vi "ChipKit Stepper Motor.vi"() -> ()   [LabVIEW 2011, in "LabVIEW Interface for ChipKit.lvlib"]
doc: "This example shows how to use the ChipKit's Stepper Motor API. The fritzing diagram shows use with the EasyStepper 4.3 or 4.4 motor controller."
uses:
  vi.lib/LabVIEW Interface for ChipKit/LabVIEW Interface for ChipKit.lvlib
panel:
  in  "VISA resource name":refnum<visa-resource-name>
  in  "Stop":bool
  in  "Stepper #":u8=1
  in  "OK Button":bool
  in  "Set Acceleration (0 to disable)":i16
  in  "# of Steps to Move":i16
  in  "Set Speed (Steps per Second)":i16=100
  out "Steps Remaining?":bool
  in  "Dial":i16(knob) scale=0.0..200.0
  in  "error in":errorcluster
  # "Preset Movement"
  # "Interactive Movement"
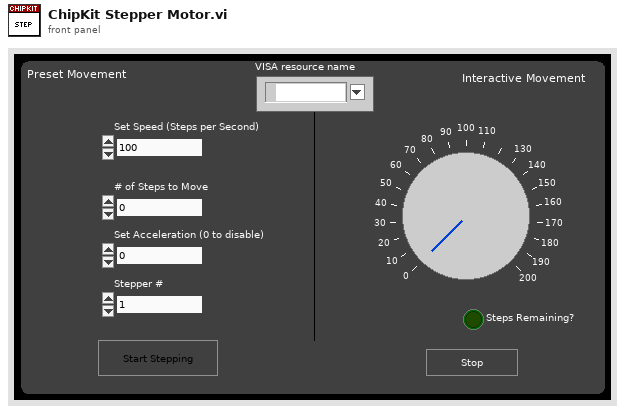
[diagram p1: front panel]
types:
  T1 = typedef "LabVIEW Interface for ChipKit.lvlib/Chipkit Resource.ctl" = cluster{"VISA resource":refnum<visa-resource-name>, "Board Type":T2, "Connection Type":enum8{"USB / Serial"}, "Bytes Per Packet (15)":u8}
  T2 = typedef "LabVIEW Interface for ChipKit.lvlib/Board Type.ctl" = enum16{"Arduino Uno", "Dimuelanove w/Atmega 328", "Mega 2560", "Chipkit Uno32", "Chipkit Max32"}
  T3 = typedef "LabVIEW Interface for ChipKit.lvlib/Chipkit Resource.ctl" = cluster{"COM Port":refnum<visa-resource-name>, "Board Type":T4, "Connection Type":T5, "Baud Rate (115200)":u32, "Bytes Per Packet (15)":u32}
  T4 = typedef "LabVIEW Interface for ChipKit.lvlib/Board Type.ctl" = enum16{"ChipKit uC32", "ChipKit Uno32", "ChipKit Max32"}
  T5 = typedef "LabVIEW Interface for ChipKit.lvlib/Connection Type.ctl" = enum8{"USB / Serial", "XBEE", "BlueSmirf (Bluetooth)"}
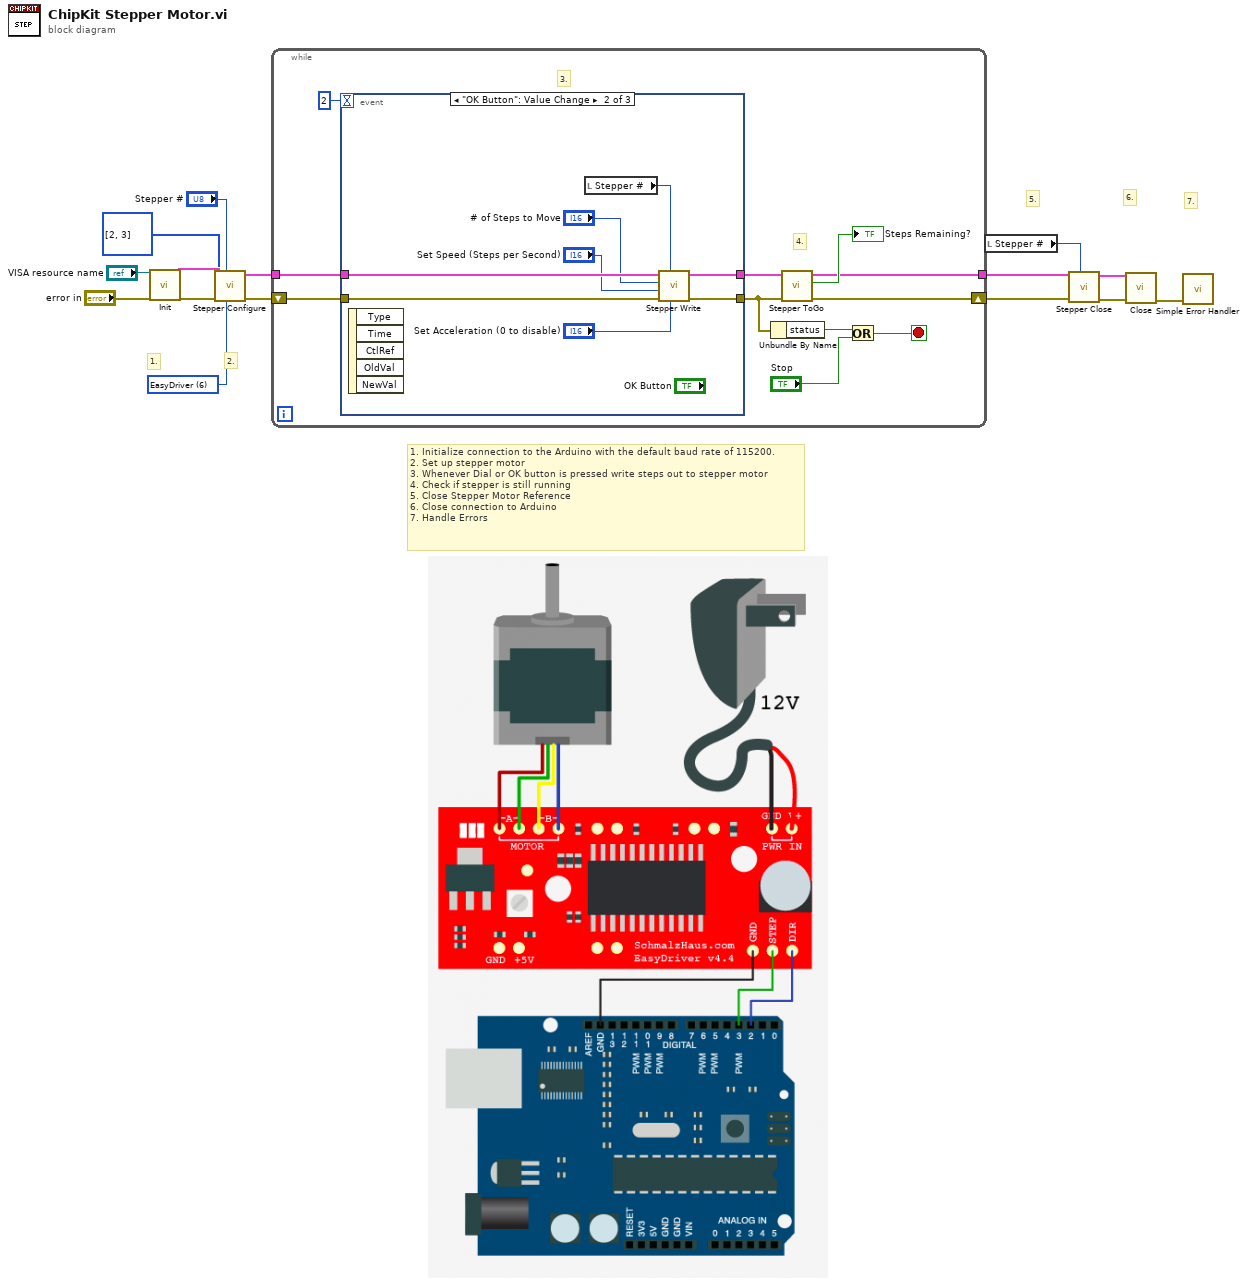
[diagram p0: block diagram]
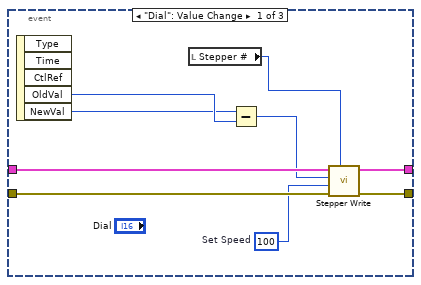
[diagram p2: hidden frame]
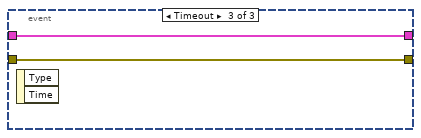
[diagram p3: hidden frame]
diagram:
  w2 = u8 6 items=["2 Wire (Pulse & Direction)"=1, "2 Wire"=2, "4 Wire"=4, "EasyDriver"=6, "AF Motor Shield (Stepper 1 & 2 Only)"=5] ("Control Method")
  # "7."
  # "6."
  # "5."
  # "2."
  # "1."
  # "1. Initialize connection to the Arduino with the default baud rate of 115200.\n2. Set up stepper motor\n3. Whenever Dial or OK button is pressed write steps out to stepper motor\n4. Check if stepper is still running\n5. Close Stepper Motor Reference \n6. Close connection to Arduino\n7. Handle Errors"
  n1 = call "Init.vi"("VISA resource"="VISA resource name", "error in"="error in") -> ("Arduino Resource"=w5:T1, "error out"=w4:errorcluster)  [unwired: 16 in]
  n2 = call "Stepper Configure.vi"("Control Method"=w2, "Stepper #"="Stepper #", "error in"=w4, "Stepper Pins"=u8[] [2, 3], "Arduino Resource"=w5) -> ("error out"=w13:errorcluster, "Arduino Resource Out"=w14:T3)  [unwired: 5 in]
  n3 = while {
    tunnel: w14 -> [w25]
    tunnel: [w19] -> w12
    shift-right: [w17] -> w11
    shift-left: w13 -> [w26]
    stop <- w23 stop-if-true
    # "4."
    # "3."
    n4 = event shown="[1] \"OK Button\": Value Change" {
      selector: _ -> [_ _ _]
      dyn-events: _ -> [_ _ _]
      timeout: 2 -> [_ _ _]
      tunnel: w26 -> [w35 w42 w44]
      tunnel: w25 -> [w34 w40 w45]
      tunnel: [w33 w41 w45] -> w21
      tunnel: [w32 w43 w44] -> w18
      event "Dial": Value Change {
        w29 = i16 100  # Set Speed
        n5 = event-data() -> ("OldVal"=w31:i16, "NewVal"=w30:i16)  [unwired: 1 in, 3 out]
        n6 = local read "Stepper #"() -> (w27:u8)
        n7 = Subtract(x=w30, y=w31) -> (x-y=w28:i16)
        n8 = call "Stepper Write.vi"("Stepper #"=w27, "error in"=w35, "Set Speed (Steps per Second)"=w29, "# of Steps to Move"=w28, "Arduino Resource"=w34) -> ("error out"=w32:errorcluster, "Arduino Resource Out"=w33:T3)  [unwired: 5 in]
      }
      event "OK Button": Value Change {
        n9 = event-data() -> ()  [unwired: 1 in, 5 out]
        n10 = local read "Stepper #"() -> (w36:u8)
        n11 = call "Stepper Write.vi"("Set Acceleration (0 to disable)"="Set Acceleration (0 to disable)", "Stepper #"=w36, "error in"=w42, "Set Speed (Steps per Second)"="Set Speed (Steps per Second)", "# of Steps to Move"="# of Steps to Move", "Arduino Resource"=w40) -> ("error out"=w43:errorcluster, "Arduino Resource Out"=w41:T3)  [unwired: 4 in]
      }
      event Timeout {
        n12 = event-data() -> ()  [unwired: 1 in, 2 out]
      }
    }
    n13 = Unbundle By Name(w18) -> ("status"=w22:bool)
    n14 = call "Stepper ToGo.vi"("error in"=w18, "Arduino Resource"=w21) -> ("error out"=w17:errorcluster, "Steps Remaining?"=→"Steps Remaining?":bool, "Arduino Resource Out"=w19:T3)  [unwired: 6 in, 1 out]
    n15 = Or(x=w22, y="Stop") -> (x .or. y?=w23:bool)
  }
  n16 = local read "Stepper #"() -> (w6:u8)
  n17 = call "Stepper Close.vi"("Stepper #"=w6, "error in"=w11, "Arduino Resource"=w12) -> ("error out"=w10:errorcluster, "Arduino Resource Out"=w9:T3)  [unwired: 7 in]
  n18 = call "Close.vi"("Arduino Resource"=w9, "error in"=w10) -> ("error out"=w15:errorcluster)  [unwired: 13 in]
  n19 = call <vilib>:"Simple Error Handler.vi"("error in (no error)"=w15) -> ()  [unwired: 4 in, 5 out]
